vi "Puff_using_Arduino.vi"() -> (5 "Plug in titles":string[](array[string]), 7 "Plug in values":string[](array[string]))   [LabVIEW 2012]
uses:
  Controls/Post_Process.ctl
  Controls/Setup.ctl
  Globals/Meas_global.vi
panel:
  out "Puff Time used":dbl=1.0 format="%.2g"
  out "EnFlo_Tunnel Metadata:Puff_duration:Sec":dbl=1.0 format="%.2g"
  out "Case Currently On":string="Loop"
  # "Change this value via the ADAM Scan Table"
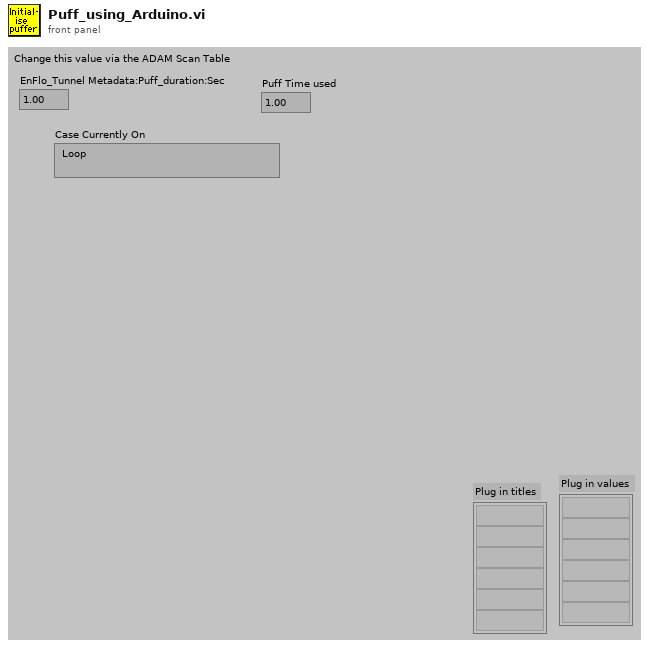
[diagram p1: front panel]
types:
  T1 = typedef "Setup.ctl" = enum16{"Run Program", "Show Setup", "Save Current Setup", "Setup Front Panel"}
  T2 = typedef "Post_Process.ctl" = enum16{"Take New Data", "Post Process Raw Data File"}
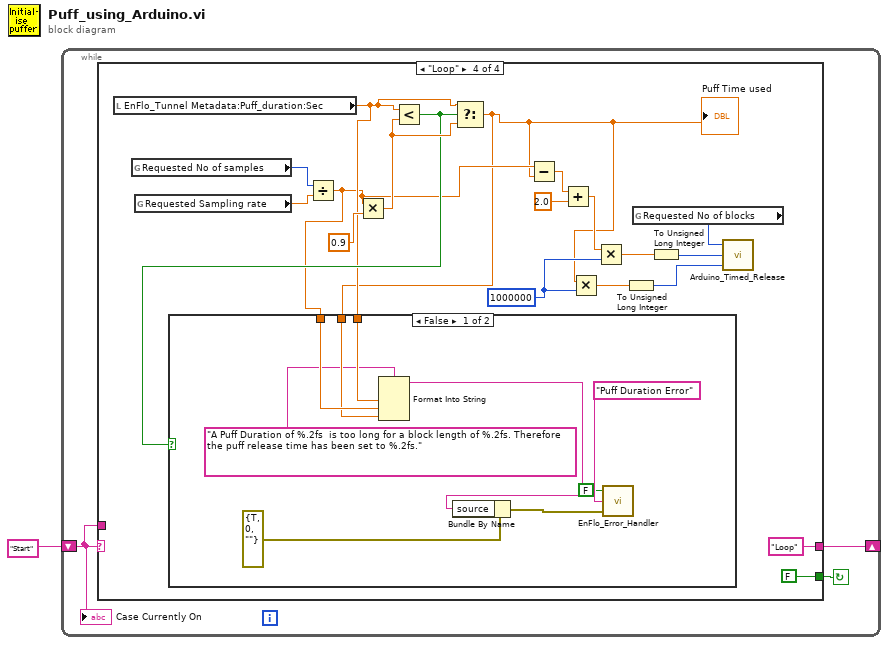
[diagram p0: block diagram]
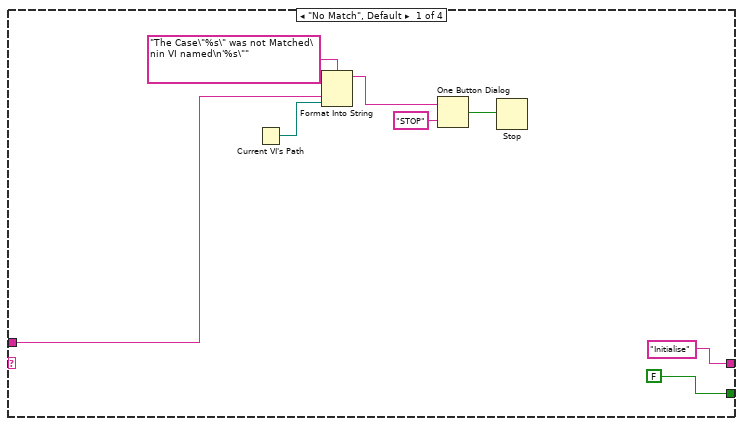
[diagram p2: hidden frame]
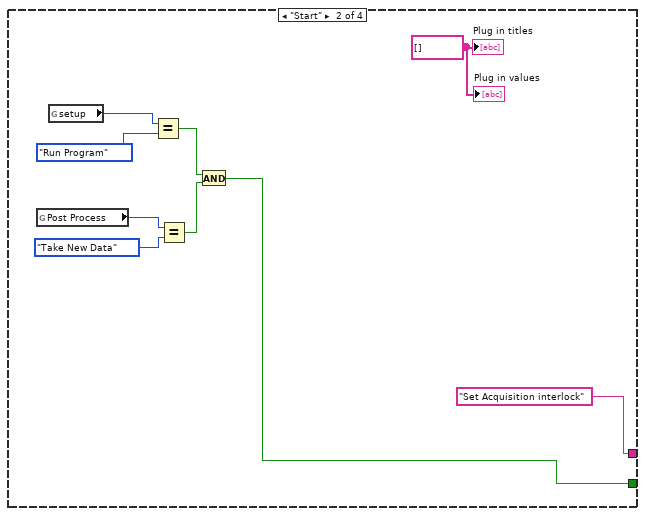
[diagram p3: hidden frame]
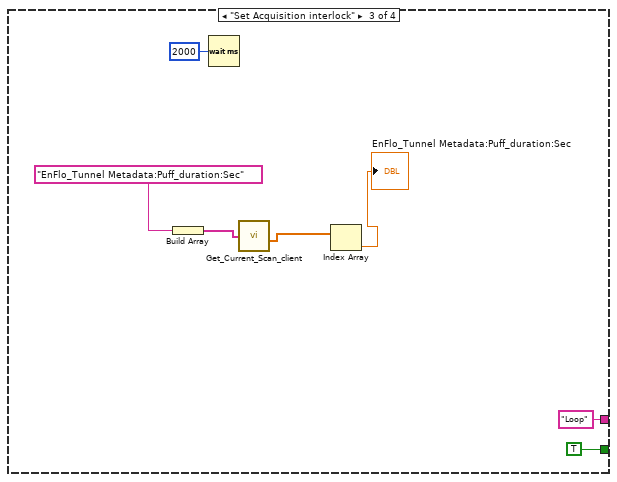
[diagram p4: hidden frame]
diagram:
  n1 = while {
    shift-left: "Start" -> [w2]
    shift-right: [w3] -> _
    stop <- w4 continue-if-true
    n2 = case shown="\"Loop\"" w2 {
      tunnel: [FALSE w13 TRUE ("Command Found") FALSE ("Command Found")] -> w4
      tunnel: ["Initialise" "Set Acquisition interlock" "Loop" "Loop"] -> w3
      tunnel: w2 -> [w7 _ _ _]
      frame "No Match", Default {
        n3 = Current VI's Path() -> (path=w6:path)
        n4 = Format Into String(format string="The Case\"%s\" was not Matched\nin VI named\n'%s\"" ("Format String"), w7, w6) -> (resulting string=w10:string)  [unwired: 2 in, 1 out]
        n5 = One Button Dialog(message=w10, button name ("OK")="STOP") -> (true=w8:bool)
        n6 = Stop(stop? (T)=w8) -> ()
      }
      frame "Start" {
        w20 = string[] [] ("Plug in titles")
        n7 = global read "Meas_global.vi" "Post Process"() -> (w15:T2)
        n8 = global read "Meas_global.vi" "setup"() -> (w14:T1)
        n9 = Equal?(x=w14, y=Setup."Run Program") -> (x = y?=w19:bool)
        n10 = Equal?(x=w15, y=Post_Process."Take New Data" ("Post Process")) -> (x = y?=w18:bool)
        n11 = And(x=w19, y=w18) -> (x .and. y?=w13:bool)
        "Plug in values" <- w20
        "Plug in titles" <- w20
      }
      frame "Set Acquisition interlock" {
        n12 = Build Array("EnFlo_Tunnel Metadata:Puff_duration:Sec") -> (w24:string[])
        n13 = Wait (ms)(milliseconds to wait=u32 2000) -> ()  [unwired: 1 out]
        n14 = call "Get_Current_Scan_client.vi"("ADAM Ch Names"=w24) -> ("Numerical Values"=w23:dbl[])  [unwired: 1 in, 2 out]
        n15 = Index Array(array=w23) -> (element=→"EnFlo_Tunnel Metadata:Puff_duration:Sec":dbl)  [unwired: 1 in]
      }
      frame "Loop" {
        w38 = u32 1000000 ("y")
        n16 = local read "EnFlo_Tunnel Metadata:Puff_duration:Sec"() -> (w32:dbl)
        n17 = global read "Meas_global.vi" "Requested No of samples"() -> (w45:i32)
        n18 = global read "Meas_global.vi" "Requested Sampling rate"() -> (w31:dbl)
        n19 = Divide(x=w45, y=w31) -> (x/y=w30:dbl)
        n20 = Multiply(x=w30, y=0.9) -> (x*y=w43:dbl)
        n21 = Less?(x=w32, y=w43) -> (x < y?=w33:bool)
        n22 = Select(t=w32, s=w33, f=w43) -> (s? t:f=w29:dbl)
        "Puff Time used" <- w29
        n23 = case shown="False" w33 {
          tunnel: w32 -> [w54 _]
          tunnel: w30 -> [w53 _]
          tunnel: w29 -> [w52 _]
          frame False {
            n24 = Format Into String(format string="A Puff Duration of %.2fs  is too long for a block length of %.2fs. Therefore the puff release time has been set to %.2fs.", w54, w53, w52) -> (resulting string=w50:string)  [unwired: 2 in, 1 out]
            n25 = Bundle By Name(cluster=errorcluster {"status"=TRUE, "code"=0, "source"=""} ("error in (no error)"), "source"=w50) -> (w55:errorcluster)
            n26 = call "EnFlo_Error_Handler.vi"("error in (no error)"=w55, "Error Type"="Puff Duration Error", "Dialog Box (T)"=FALSE) -> ()  [unwired: 3 out]
          }
          frame True {
          }
        }
        n27 = Subtract(x=w30, y=w29) -> (x-y=w36:dbl)
        n28 = Add(x=w36, y=2.0) -> (x+y=w34:dbl)
        n29 = Multiply(x=w29, y=w38) -> (x*y=w41:dbl)
        n30 = Multiply(x=w34, y=w38) -> (x*y=w39:dbl)
        n31 = To Unsigned Long Integer(number=w41) -> (unsigned 32bit integer=w40:u32)
        n32 = global read "Meas_global.vi" "Requested No of blocks"() -> (w42:i32)
        n33 = To Unsigned Long Integer(number=w39) -> (unsigned 32bit integer=w37:u32)
        n34 = call "Arduino_Timed_Release.vi"("Time to hold source ON (microseconds)"=w40, "Time to hold source OFF (microseconds)"=w37, "Number of cycles"=w42) -> ()  [unwired: 2 out]
      }
    }
    "Case Currently On" <- w2
  }
